vi "To JSON Tree.vi"(8 "error in (no error)":errorcluster, 11 "id in":refnum<class "id.lvclass">) -> (0 "error out":errorcluster, 2 "JSON out":refnum<class "JSON Datatype.lvclass">, 3 "id out":refnum<class "id.lvclass">)   [LabVIEW 2015, in "id.lvclass"]
uses:
  id.lvclass
  <vilib>/National Instruments/JSON Support for LabVIEW/JSON Data Classes/JSON Datatype/JSON Datatype.lvclass
  id.lvclass/id.ctl
  <vilib>/National Instruments/JSON Support for LabVIEW/JSON Parsing/Tokenize  JSON String.vi
  <vilib>/Utility/error.llb/Trim Whitespace.vi
  <vilib>/National Instruments/JSON Support for LabVIEW/JSON Data Classes/JSON Datatype/New JSON.vi
  <vilib>/National Instruments/JSON Support for LabVIEW/JSON Data Classes/JSON Numeric/New JSON Numeric.vi
  <vilib>/National Instruments/JSON Support for LabVIEW/JSON Data Classes/JSON Boolean/New JSON Boolean.vi
  <vilib>/National Instruments/JSON Support for LabVIEW/JSON Data Classes/JSON Null/New JSON Null.vi
  <vilib>/National Instruments/JSON Support for LabVIEW/JSON Parsing/Tokens to String.vi
  <vilib>/National Instruments/JSON Support for LabVIEW/JSON Data Classes/JSON String/New JSON String.vi
  <vilib>/National Instruments/JSON Support for LabVIEW/JSON Parsing/Tokens to Array.vi
  <vilib>/National Instruments/JSON Support for LabVIEW/JSON Parsing/Tokens to Object.vi
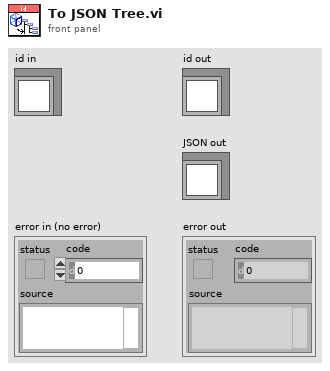
[diagram p1: front panel]
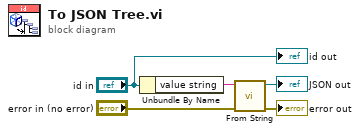
[diagram p0: block diagram]
diagram:
  n1 = Unbundle By Name("id in") -> ("value string"=w4:string)
  n2 = call <vilib>:"From String.vi"("error in (no error)"="error in (no error)", "JSON String"=w4) -> ("error out"=→"error out":errorcluster, "JSON out"=→"JSON out":refnum<class "JSON Datatype.lvclass">)  [unwired: 8 in]
  "id out" <- "id in"
